vi "Filter lines.vi"(4 "max dist":dbl, 5 "LRF pos":dbl[](array[numeric]), 6 "P2y":dbl[](array[numeric]), 7 "P1y":dbl[](array[numeric]), 8 "P2x":dbl[](array[numeric]), 9 "P1x":dbl[](array[numeric])) -> (0 "P2y new":dbl[](array[numeric]), 1 "P1y new":dbl[](array[numeric]), 2 "P2x new":dbl[](array[numeric]), 3 "P1x new":dbl[](array[numeric]))   [LabVIEW 2009]
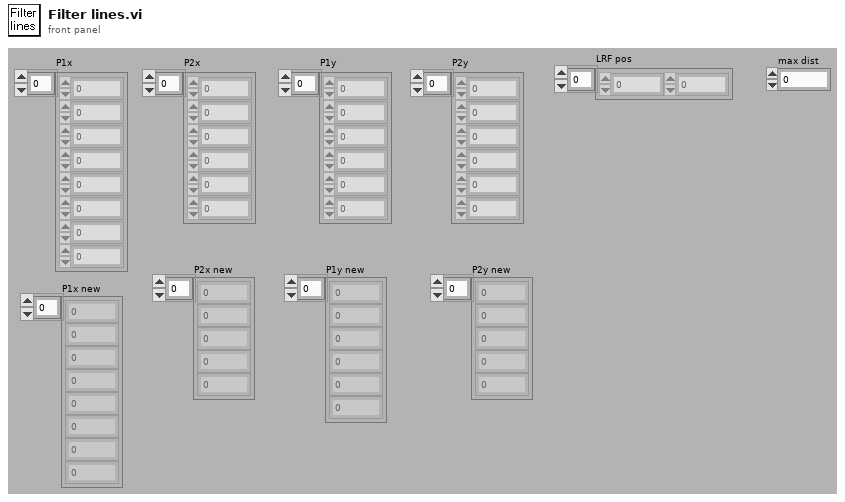
[diagram p1: front panel]
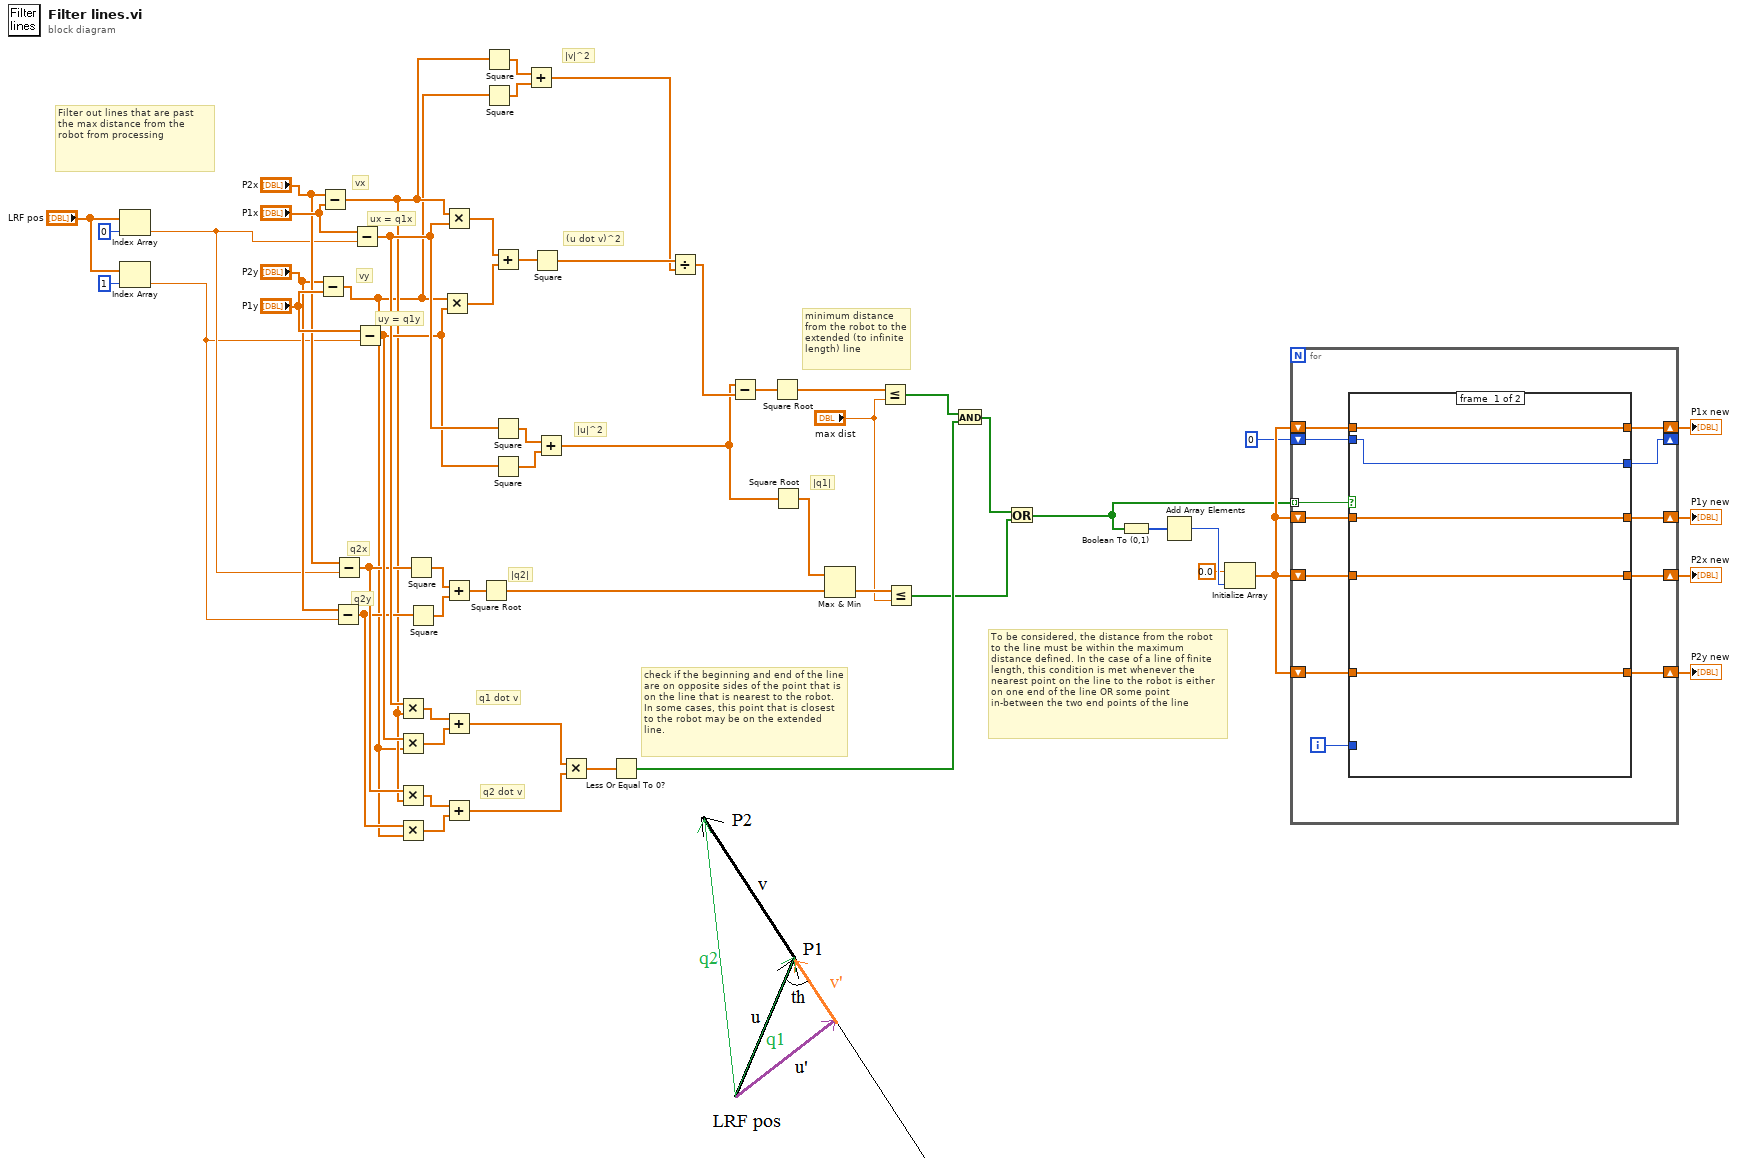
[diagram p0: block diagram]
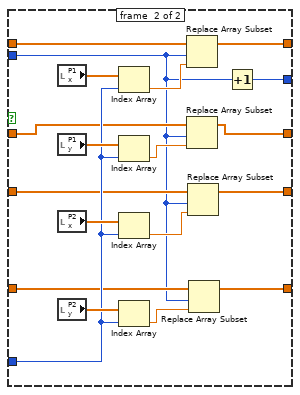
[diagram p2: hidden frame]
diagram:
  # "To be considered, the distance from the robot to the line must be within the maximum distance defined. In the case of a line of finite length, this condition is met whenever the nearest point on the line to the robot is either on one end of the line OR some point in-between the two end points of the line"
  # "|q1|"
  # "check if the beginning and end of the line are on opposite sides of the point that is on the line that is nearest to the robot. In some cases, this point that is closest to the robot may be on the extended line."
  # "q2 dot v"
  # "q1 dot v"
  # "q2y"
  # "q2x"
  # "|q2|"
  # "Filter out lines that are past the max distance from the robot from processing"
  # "minimum distance from the robot to the extended (to infinite length) line"
  # "|v|^2"
  # "|u|^2"
  # "(u dot v)^2"
  # "uy = q1y"
  # "ux = q1x"
  # "vy"
  # "vx"
  n1 = Index Array(array="LRF pos", index=0) -> (element=w28:dbl)
  n2 = Index Array(array="LRF pos", index=1) -> (element=w27:dbl)
  n3 = Subtract(x="P2y", y="P1y") -> (x-y=w11:dbl[])
  n4 = Subtract(x="P2x", y="P1x") -> (x-y=w12:dbl[])
  n5 = Subtract(x="P2y", y=w27) -> (x-y=w13:dbl[])
  n6 = Subtract(x="P2x", y=w28) -> (x-y=w14:dbl[])
  n7 = Subtract(x="P1x", y=w28) -> (x-y=w20:dbl[])
  n8 = Subtract(x="P1y", y=w27) -> (x-y=w19:dbl[])
  n9 = Multiply(x=w20, y=w12) -> (x*y=w18:dbl[])
  n10 = Multiply(x=w19, y=w11) -> (x*y=w17:dbl[])
  n11 = Multiply(x=w14, y=w12) -> (x*y=w16:dbl[])
  n12 = Multiply(x=w13, y=w11) -> (x*y=w15:dbl[])
  n13 = Square(x=w14) -> (x^2=w26:dbl[])
  n14 = Square(x=w13) -> (x^2=w25:dbl[])
  n15 = Multiply(x=w11, y=w19) -> (x*y=w50:dbl[])
  n16 = Multiply(x=w12, y=w20) -> (x*y=w51:dbl[])
  n17 = Add(x=w26, y=w25) -> (x+y=w24:dbl[])
  n18 = Add(x=w18, y=w17) -> (x+y=w10:dbl[])
  n19 = Add(x=w16, y=w15) -> (x+y=w9:dbl[])
  n20 = Square Root(x=w24) -> (sqrt(x)=w22:dbl[])
  n21 = Square(x=w12) -> (x^2=w46:dbl[])
  n22 = Square(x=w11) -> (x^2=w45:dbl[])
  n23 = Add(x=w51, y=w50) -> (x+y=w47:dbl[])
  n24 = Square(x=w20) -> (x^2=w49:dbl[])
  n25 = Square(x=w19) -> (x^2=w48:dbl[])
  n26 = Add(x=w46, y=w45) -> (x+y=w43:dbl[])
  n27 = Square(x=w47) -> (x^2=w44:dbl[])
  n28 = Add(x=w49, y=w48) -> (x+y=w31:dbl[])
  n29 = Multiply(x=w10, y=w9) -> (x*y=w8:dbl[])
  n30 = Less Or Equal To 0?(x=w8) -> (x <= 0?=w7:bool[])
  n31 = Divide(x=w44, y=w43) -> (x/y=w42:dbl[])
  n32 = Subtract(x=w31, y=w42) -> (x-y=w41:dbl[])
  n33 = Square Root(x=w41) -> (sqrt(x)=w21:dbl[])
  n34 = Square Root(x=w31) -> (sqrt(x)=w23:dbl[])
  n35 = Max & Min(x=w23, y=w22) -> (min(x,y)=w5:dbl[])  [unwired: 1 out]
  n36 = Less Or Equal?(x=w21, y="max dist") -> (x <= y?=w6:bool[])
  n37 = Less Or Equal?(x=w5, y="max dist") -> (x <= y?=w3:bool[])
  n38 = And(x=w6, y=w7) -> (x .and. y?=w2:bool[])
  n39 = Or(x=w2, y=w3) -> (x .or. y?=w1:bool[])
  n40 = Boolean To (0,1)(Boolean=w1) -> (0, 1=w40:i16[])
  n41 = Add Array Elements(numeric array=w40) -> (sum=w39:i16)
  n42 = Initialize Array(0.0 ("element"), w39) -> (w37:dbl[])
  n43 = for {
    tunnel: w1 -> [w68] mode=indexing
    shift-right: [w63] -> w35
    shift-left: w37 -> [w66]
    shift-right: [w61] -> w34
    shift-left: w37 -> [w62]
    shift-right: [w59] -> w33
    shift-left: w37 -> [w60]
    shift-right: [w57] -> w32
    shift-left: w37 -> [w58]
    shift-right: [w64] -> _
    shift-left: 0 -> [w65]
    i -> [w67]
    n44 = case shown="True" w68 {
      tunnel: w67 -> [_ w88]
      tunnel: w66 -> [w72 w86]
      tunnel: w65 -> [w73 w75]
      tunnel: [w73 w87] -> w64
      tunnel: [w72 w84] -> w63
      tunnel: w62 -> [w71 w83]
      tunnel: [w71 w82] -> w61
      tunnel: w60 -> [w70 w80]
      tunnel: [w70 w79] -> w59
      tunnel: w58 -> [w69 w77]
      tunnel: [w69 w76] -> w57
      frame #0 {
      }
      frame #1 {
        n45 = local read "P1x"() -> (w92:dbl[])
        n46 = local read "P1y"() -> (w91:dbl[])
        n47 = local read "P2x"() -> (w90:dbl[])
        n48 = local read "P2y"() -> (w89:dbl[])
        n49 = Index Array(array=w92, index=w88) -> (element=w85:dbl)
        n50 = Index Array(array=w91, index=w88) -> (element=w81:dbl)
        n51 = Index Array(array=w90, index=w88) -> (element=w78:dbl)
        n52 = Index Array(array=w89, index=w88) -> (element=w74:dbl)
        n53 = Replace Array Subset(array=w86, new element=w85, index=w75) -> (w84:dbl[])
        n54 = Replace Array Subset(array=w83, new element=w81, index=w75) -> (w82:dbl[])
        n55 = Replace Array Subset(array=w80, new element=w78, index=w75) -> (w79:dbl[])
        n56 = Replace Array Subset(array=w77, new element=w74, index=w75) -> (w76:dbl[])
        n57 = Increment(x=w75) -> (x+1=w87:i32)
      }
    }
  }
  "P1x new" <- w35
  "P1y new" <- w34
  "P2x new" <- w33
  "P2y new" <- w32
